vi "Test App Set and Get Process From Branch.vi"(8 "error in (no error)":errorcluster, 11 "Application Test in":refnum<class "Application Dev Test.lvclass">) -> (0 "error out":errorcluster, 3 "Application Test out":refnum<class "Application Dev Test.lvclass">)   [LabVIEW 2020, in "Application Dev Test.lvclass"]
uses:
  Application Dev Test.lvclass
  C:/Program Files (x86)/National Instruments/LabVIEW 2020/vi.lib/Astemes/LUnit/Test Case.lvclass
  source/Framework/Process/Process.lvclass
  source/Framework/Process/Process.lvclass/Process.ctl
  source/Framework/Application/Application.lvclass/Application.ctl
  <vilib>/Astemes/LUnit/Test Case.lvclass/Test Case.ctl
  <vilib>/Astemes/LUnit/LUnit Assertion Result.lvclass/LUnit Assertion Result.ctl
  <vilib>/Astemes/LUnit/LUnit Test Case Result.lvclass/LUnit Test Case Result.ctl
  <vilib>/Astemes/LUnit/LUnit Method Result.lvclass/LUnit Method Result.ctl
  source/Framework/Application/Private/Add Process to Map.vi
  source/Framework/Application/Private/Start Idle Processes if Running.vi
  source/Framework/Application/Private/Throw Error If Process Already in App.vi
  source/Framework/Process/Protected/Messaging/Enqueue Message.vi
  source/Framework/Process/Public/Lifecycle/Get Lifecycle State.vi
  source/Framework/Process/Protected/SubVIs/Set Context.vi
  source/Framework/Application/Private/Retrieve Process from App.vi
  source/Framework/Application/Private/Parse Process Name.vi
  source/Framework/Application/Private/Get Process from Map.vi
  source/Framework/Process/Protected/Messaging/Request Message.vi
  <vilib>/Astemes/LUnit/Palette/Fail.vi
  <vilib>/Astemes/LUnit/Palette/Pass.vi
  <vilib>/Astemes/LUnit/Set Assertion Type.vi
  source/Framework/Process/Private/SubVIs/Wait for finish.vi
  source/Framework/Process/Private/SubVIs/Set Lifecycle State.vi
  source/Framework/Process/Private/SubVIs/Handle Debug Data.vi
  <vilib>/Utility/error.llb/Clear Errors.vi
  source/Framework/Process/Public/Lifecycle/Leave Process Loop.vi
  <vilib>/AdvancedString/Delimited String to 1D String Array.vi
  source/Framework/Process/Private/SubVIs/Enqueue Request Message.vi
  <vilib>/Astemes/LUnit/Add test result.vi
  <vilib>/Astemes/LUnit/LUnit Write Passed.vi
  <vilib>/Astemes/LUnit/LUnit Write Message.vi
  <vilib>/Astemes/LUnit/LUnit Write Description.vi
  <vilib>/Astemes/LUnit/LUnit Write Assertion Type.vi
  source/Framework/Logging/Log Debug.vi
  <vilib>/AdvancedString/1D String Array to Delimited String.vi
  <vilib>/Utility/High Resolution Relative Seconds.vi
  <vilib>/Astemes/LUnit/LUnit Record Assertion Result.vi
  <vilib>/Astemes/LUnit/LUnit Aggregate Assertion Results.vi
  <vilib>/Astemes/LUnit/Assertion Result/LUnit Read Status.vi
  <vilib>/Astemes/LUnit/LUnit Read Message.vi
  <vilib>/Astemes/LUnit/LUnit Read Description.vi
  <vilib>/Astemes/LUnit/Method Result/LUnit Merge Status.vi
  <vilib>/Astemes/LUnit/LUnit Concatenate result strings.vi
  source/Framework/Application/Application.lvclass
  C:/Git/astemes-triarc-framework/source/Framework/Process/Process.lvclass
  <vilib>/Utility/error.llb/Error Cluster From Error Code.vi
  source/Framework/Process/Private/SubVIs/Wait for Response Message.vi
  <vilib>/Astemes/LUnit/LUnit Assertion Result.lvclass
  <vilib>/Astemes/LUnit/Test Case.lvclass
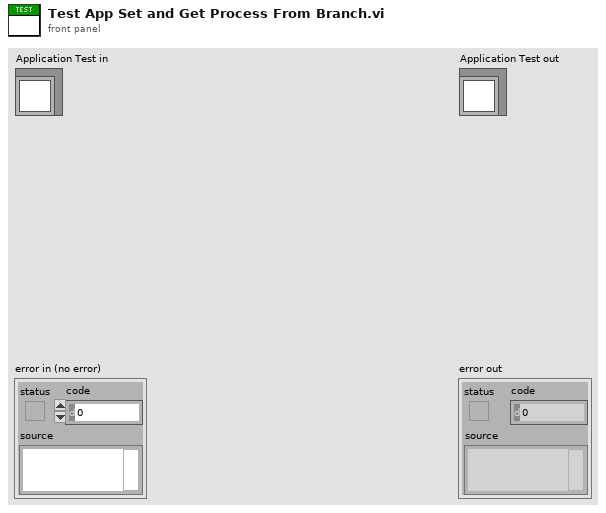
[diagram p1: front panel]
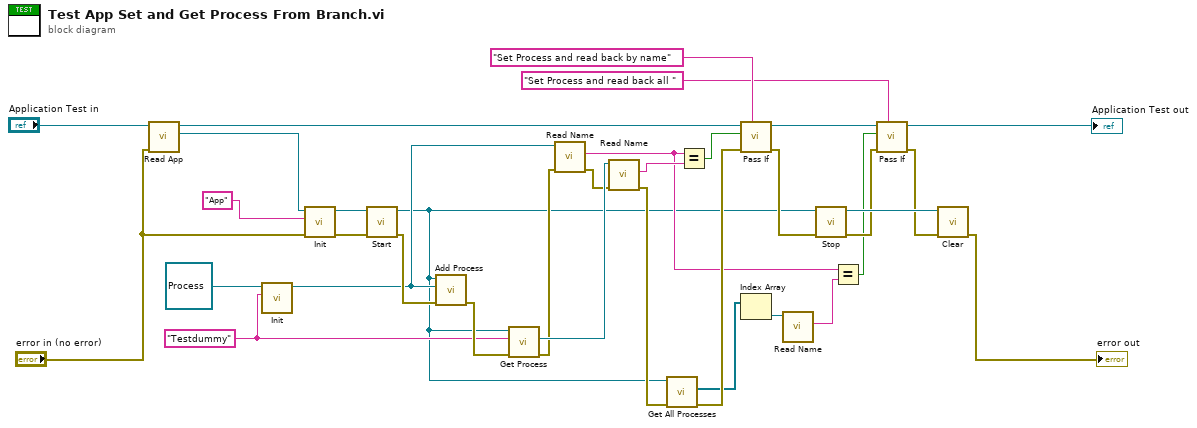
[diagram p0: block diagram]
diagram:
  w12 = "Testdummy" ("Name")
  n1 = call "Read App.vi"("error in (no error)"="error in (no error)", "Application Test In"="Application Test in") -> ("App out"=w33:refnum<class "Application.lvclass">, "Application Test Out"=w34:refnum<class "Application Dev Test.lvclass">)  [unwired: 7 in, 1 out]
  n2 = call-dynamic "Init.vi"("Name"=w12, "Process In"=refnum<class "Process.lvclass"> refnum ("Process.lvclass")) -> ("Process Out"=w7:refnum<class "Process.lvclass">)  [unwired: 8 in, 1 out]
  n3 = call-dynamic "Init.vi"("error in (no error)"="error in (no error)", "Name"="App", "Process In"=w33) -> ("error out"=w31:errorcluster, "Process Out"=w32:refnum<class "Application.lvclass">)  [unwired: 7 in]
  n4 = call "Start.vi"("error in (no error)"=w31, "Process In"=w32) -> ("error out"=w28:errorcluster, "Process Out"=w1:refnum<class "Application.lvclass">)  [unwired: 7 in, 1 out]
  n5 = call "Add Process.vi"("error in (no error)"=w28, "Process"=w7, "Application In"=w1) -> ("error out"=w29:errorcluster)  [unwired: 7 in, 1 out]
  n6 = call "Get Process.vi"("error in (no error)"=w29, "Process Name"=w12, "Application In"=w1) -> ("error out"=w3:errorcluster, "App Process"=w25:refnum<class "Process.lvclass">)  [unwired: 6 in, 1 out]
  n7 = call "Read Name.vi"("error in (no error)"=w3, "Process In"=w7) -> ("error out"=w4:errorcluster, "Qualified Name"=w6:string)  [unwired: 6 in, 2 out]
  n8 = call "Read Name.vi"("error in (no error)"=w4, "Process In"=w25) -> ("error out"=w2:errorcluster, "Qualified Name"=w8:string)  [unwired: 6 in, 2 out]
  n9 = call "Get All Processes.vi"("error in (no error)"=w2, "Application In"=w1) -> ("error out"=w23:errorcluster, "App Processes"=w21:refnum<class "Process.lvclass">[])  [unwired: 7 in, 1 out]
  n10 = Equal?(x=w6, y=w8) -> (x = y?=w24:bool)
  n11 = call <vilib>:"Pass If.vi"("Description"="Set Process and read back by name", "error in (no error)"=w23, "Pass?"=w24, "LUnit Test Case In"=w34) -> ("error out"=w22:errorcluster, "LUnit Test Case Out"=w26:refnum<class "Application Dev Test.lvclass">)  [unwired: 6 in]
  n12 = Index Array(array=w21) -> (element=w20:refnum<class "Process.lvclass">)  [unwired: 1 in]
  n13 = call "Read Name.vi"("Process In"=w20) -> ("Qualified Name"=w5:string)  [unwired: 7 in, 3 out]
  n14 = call "Stop.vi"("error in (no error)"=w22, "Process In"=w1) -> ("error out"=w16:errorcluster, "Process Out"=w30:refnum<class "Application.lvclass">)  [unwired: 7 in, 1 out]
  n15 = Equal?(x=w6, y=w5) -> (x = y?=w14:bool)
  n16 = call <vilib>:"Pass If.vi"("Description"="Set Process and read back all ", "error in (no error)"=w16, "Pass?"=w14, "LUnit Test Case In"=w26) -> ("error out"=w15:errorcluster, "LUnit Test Case Out"=→"Application Test out":refnum<class "Application Dev Test.lvclass">)  [unwired: 6 in]
  n17 = call-dynamic "Clear.vi"("error in (no error)"=w15, "Application In"=w30) -> ("error out"=→"error out":errorcluster)  [unwired: 9 in]
